vi "FGV - Plot Management.vi"(5 "Names":cluster{string[]}[](array[cluster]), 6 "Mode":T1(ring), 7 "references in":refnum<vi>[](array[refnum]), 8 "error in (no error)":errorcluster, 10 "Values":dbl[](array[numeric])=[0.0, 1.0, 2.0, 3.0, 4.0], 11 "UUIDs":string[](array[string])) -> (0 "error out":errorcluster)   [LabVIEW 2018]
doc: "Functional global variable. Manages plots in order to link actions to change plot properties, i.e. updating values, clearing history, aligning axis properties, etc. Currently only supports plots with a 2D double numeric type."
uses:
  Core Test Control System/support/Index Array Elements/Index Array Elements - double.vi
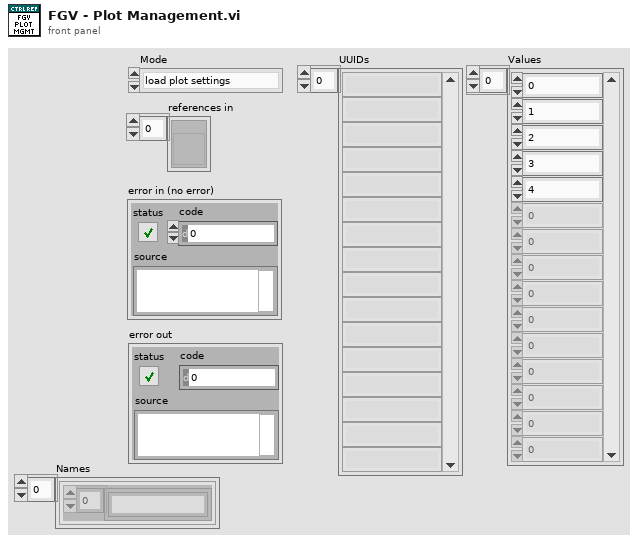
[diagram p1: front panel]
types:
  T1 = enum16{"load plot settings", "save plot settings", "update plot names", "update plot values", "clear plot histories"}
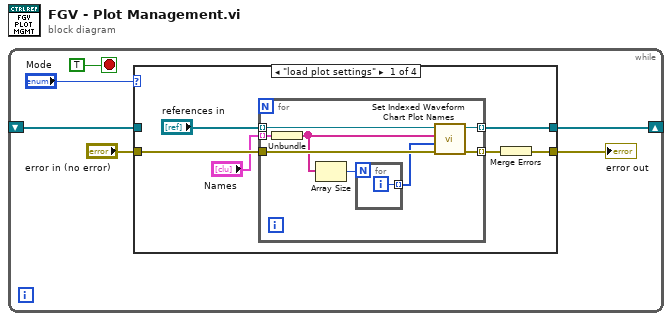
[diagram p0: block diagram]
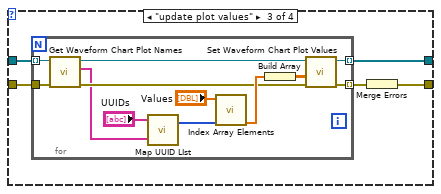
[diagram p3: hidden frame]
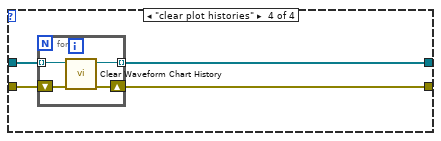
[diagram p4: hidden frame]
diagram:
  n1 = while {
    shift-right: [w4] -> _
    shift-left: _ -> [w3]
    stop <- TRUE stop-if-true
    n2 = case shown="\"load plot settings\"" "Mode" {
      tunnel: [w11 w23 w27 w43] -> w4
      tunnel: w3 -> [_ w23 w28 w44]
      tunnel: [w8 w22 w25 w42] -> w1
      tunnel: "error in (no error)" -> [w10 w22 w24 w41]
      frame "load plot settings" {
        n3 = for {
          tunnel: "references in" -> [w20] mode=indexing
          tunnel: [w19] -> w11 mode=indexing
          tunnel: w10 -> [w18]
          tunnel: [w17] -> w9 mode=indexing
          tunnel: "Names" -> [w16] mode=indexing
          n4 = Unbundle(w16) -> (w15:string[])
          n5 = Array Size(array=w15) -> (size(s)=w14:i32)
          n6 = for {
            N: w14 -> [_]
            tunnel: [w21] -> w13 mode=indexing
            i -> [w21]
          }
          n7 = call "Set Indexed Waveform Chart Plot Names.vi"("error in (no error)"=w18, "Indices"=w13, "Plot Names"=w15, "reference in"=w20) -> ("error out"=w17:errorcluster, "reference out"=w19:refnum<vi>)  [unwired: 6 in]
        }
        n8 = Merge Errors(w9) -> (w8:errorcluster)
      }
      frame Default {
      }
      frame "update plot values" {
        n9 = for {
          tunnel: w28 -> [w33] mode=indexing
          tunnel: [w34] -> w27 mode=indexing
          tunnel: [w40] -> w26 mode=indexing
          tunnel: w24 -> [w31]
          n10 = call "Get Waveform Chart Plot Names.vi"("error in (no error)"=w31, "reference in"=w33) -> ("error out"=w30:errorcluster, "Plot Names"=w29:string[], "reference out"=w32:refnum<vi>)  [unwired: 7 in]
          n11 = call "Map UUID LIst.vi"("UUIDs"=w29, "UUID List"="UUIDs") -> ("indices"=w39:i32[])  [unwired: 1 out]
          n12 = call-poly "Index Array Elements.vi"("indices (none)"=w39, "1D Array"="Values") -> ("output array"=w36:dbl[])  [unwired: 5 in]
          n13 = Build Array(w36) -> (w35:dbl[][])
          n14 = call "Set Waveform Chart Plot Values.vi"("error in (no error)"=w30, "Values"=w35, "WaveformChart in"=w32) -> ("error out"=w40:errorcluster, "WaveformChart out"=w34:refnum<vi>)  [unwired: 7 in]
        }
        n15 = Merge Errors(w26) -> (w25:errorcluster)
      }
      frame "clear plot histories" {
        n16 = for {
          tunnel: w44 -> [w48] mode=indexing
          tunnel: [w47] -> w43 mode=indexing
          shift-right: [w46] -> w42
          shift-left: w41 -> [w45]
          n17 = call "Clear Waveform Chart History.vi"("error in (no error)"=w45, "references in"=w48) -> ("error out"=w46:errorcluster, "references out"=w47:refnum<vi>)  [unwired: 8 in]
        }
      }
    }
    "error out" <- w1
  }
